vi "DAQX mod 1SDI v04.vi"(0 "resource name":refnum<k15>="PXI1Slot2", 1 "close (T)":bool=TRUE, 2 "Record Data":bool, 3 "numSamples":i32=-1, 4 "max time (s)":dbl=10.0 caption="max time", 5 "min sample rate":dbl=100000000.0, 6 "File location":path, 7 "error in":errorcluster, 8 "reference position":dbl=50.0, 9 "Additional text":string, 10 "Type of measurement":T2, 11 "Name root":string, 13 "channel parameters":T4(array[cluster])=[{"channel name"="0", "input impedance"=0, "maximum input frequency"=30000000.0, "vertical coupling"=1, "probe attenuation"=1.0, "vertical range"=2.0, "vertical offset"=0.0, "channel enabled"=TRUE}, {"channel name"="1", "input impedance"=0, "maximum input frequency"=30000000.0, "vertical coupling"=1, "probe attenuation"=1.0, "vertical range"=2.0, "vertical offset"=0.0, "channel enabled"=TRUE}] {"input impedance" items=["1 mega ohm"=0, "50 ohms"=2]; "vertical coupling" items=["AC", "DC", "Ground"]}, 15 "reset sn":bool) -> (18 "wfm out":waveform(dbl)[](array[waveform]), 22 "Parameters values file":string, 24 "actualSamples 0":i32, 26 "actualSamples 1":i32, 27 "error out":errorcluster caption="error out final")   [LabVIEW 2013]
doc: "Configures and acquires data from an NI-SCOPE high-speed digitizer.\n--------------------\n\nThis Express VI is configured as follows:\n\nDevice: PXI1Slot2 (PXI-5122)\nSample Rate (S/s): 100M\nRecord length: 2k\nAcquisition Mode: N Samples\nChannel 0\n - Range (V): 2\n - Offset (V): 0\n - Probe attenuation: 1\n - Coupling: \n - Input impedence: 1 \n - Bandwidth (Hz): 0\nChannel 1\n - Range (V): 2\n - Offset (V): 0\n - Probe attenuation: 1\n - Coupling: \n - Input impedence: 1 \n - Bandwidth (Hz): 0\nImmediate"
uses:
  <instrlib>/niScope/Controls/niScope vertical coupling.ctl
  Strict Type Defs/type_meas_enum.ctl
  <instrlib>/niScope/Controls/niScope timestamp type.ctl
  Global VIs/shotnoise.vi
  <instrlib>/niScope/Configure/Trigger/niScope Configure Trigger Immediate.vi
  <instrlib>/niScope/Acquire/Fetch/niScope Multi Fetch Binary 16.vi
  <instrlib>/niScope/Acquire/Fetch/niScope Multi Fetch WDT.vi
panel:
  out "Numeric":i32
  out "acquisition status":i32 caption="集録ステータス"
  out "Chan 1 params":T1
  out "Chan 0 params":T1
  out "file location into parameter files":path
  out "size(s)":i32
  out "actual sample rate":dbl
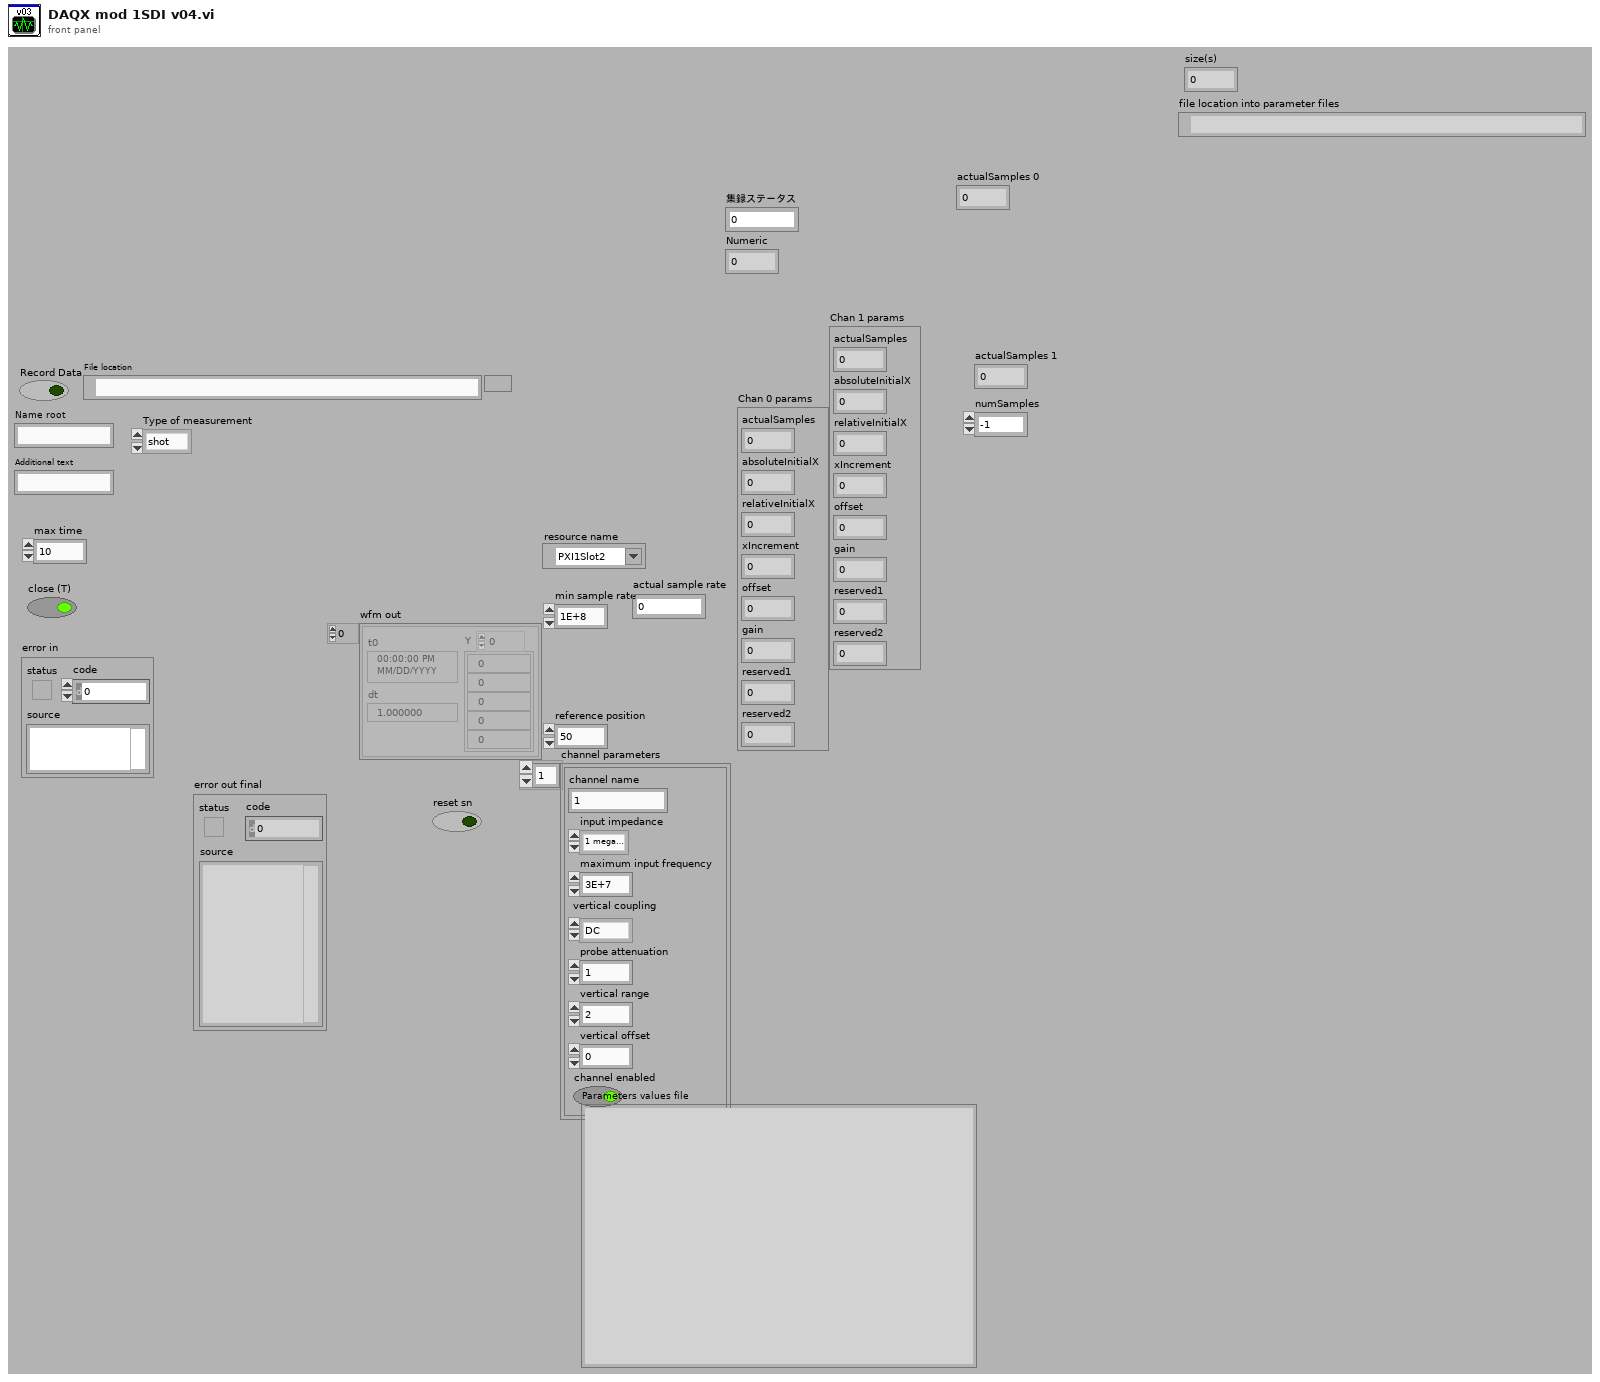
[diagram p1: front panel]
types:
  T1 = cluster{"actualSamples":i32, "absoluteInitialX":dbl, "relativeInitialX":dbl, "xIncrement":dbl, "offset":dbl, "gain":dbl, "reserved1":dbl, "reserved2":dbl}
  T2 = typedef "type_meas_enum.ctl" = enum16{"shot", "x", "p", "electronic"}
  T3 = typedef "niScope vertical coupling.ctl" = i32
  T4 = cluster{"channel name":string, "input impedance":u32, "maximum input frequency":dbl, "vertical coupling":T3, "probe attenuation":dbl, "vertical range":dbl, "vertical offset":dbl, "channel enabled":bool}[]
  T5 = typedef "niScope timestamp type.ctl" = i32
  T6 = cluster{"actualSamples":i32, "absoluteInitialX":dbl, "relativeInitialX":dbl, "xIncrement":dbl, "offset":dbl, "gain":dbl, "reserved1":dbl, "reserved2":dbl}[]
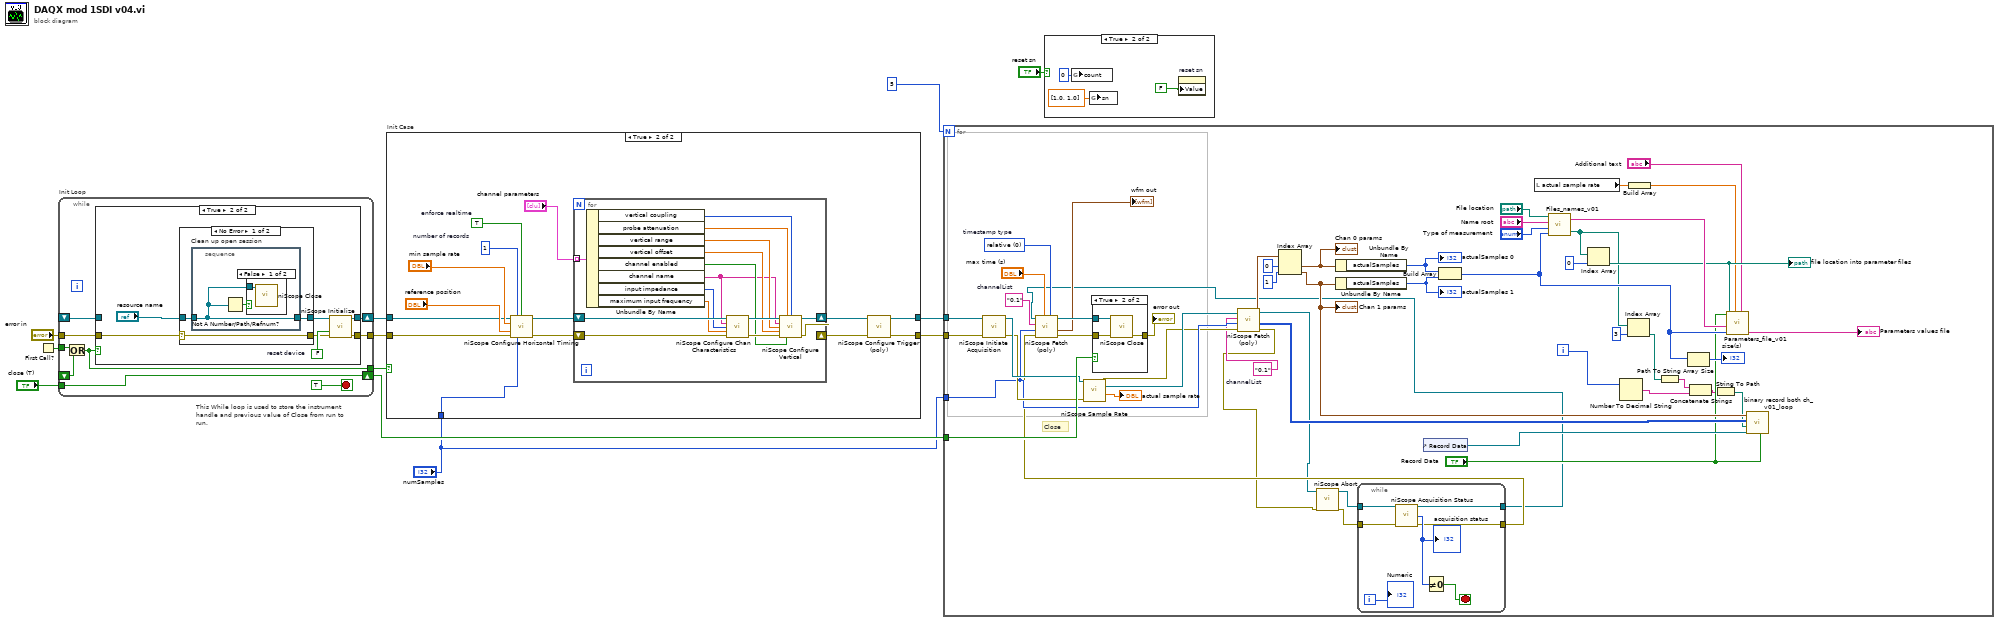
[diagram p0: block diagram]
diagram:
  # "This While loop is used to store the instrument handle and previous value of Close from run to run."
  n1 = First Call?() -> (First Call?: T/F=w10:bool)
  n2 = while "Init Loop" {
    tunnel: w10 -> [w21]
    shift-right: [w20] -> w6
    shift-left: _ -> [w17]
    tunnel: "close (T)" -> [w20]
    shift-right: [w19] -> w9
    shift-left: _ -> [w18]
    tunnel: [w15] -> w8
    tunnel: "error in" -> [w14]
    tunnel: [w13] -> w7
    stop <- TRUE ("stopInit") stop-if-true
    n3 = Or(x=w21, y=w17) -> (x .or. y?=w13:bool)
    n4 = case "Select_Init" shown="True" w13 {
      tunnel: [w23 w28] -> w19
      tunnel: w18 -> [w23 _]
      tunnel: [w22 w27] -> w15
      tunnel: w14 -> [w22 w26]
      frame False {
      }
      frame True {
        w29 = FALSE  # reset device
        n5 = case shown="No Error" w26 {
          selector: w26 -> [w31 w37]
          tunnel: [w33 w38] -> w30
          tunnel: "resource name" -> [w32 w38]
          tunnel: [w31 w37] -> w25
          frame No Error {
            n6 = stacked-sequence "Clean up open session" {
              tunnel: w32 -> [w34]
              tunnel: [w34] -> w33
              frame #0 {
                n7 = Not A Number/Path/Refnum?(number/path/refnum=w34) -> (NaN/Path/Refnum?=w35:bool)
                n8 = case shown="False" w35 {
                  tunnel: w34 -> [w36 _]
                  frame False {
                    n9 = call <instrlib>:"niScope Close.vi"("instrument handle"=w36) -> ()  [unwired: 1 in, 14 out]
                  }
                  frame True {
                  }
                }
              }
            }
          }
          frame Error {
          }
        }
        n10 = call <instrlib>:"niScope Initialize.vi"("resource name"=w30, "reset device"=w29, "error in"=w25) -> ("instrument handle"=w28:refnum<k15>, "error out"=w27:errorcluster)  [unwired: 2 in, 9 out]
      }
    }
  }
  n11 = case "Init Case" shown="True" w7 {
    tunnel: w8 -> [w39 w45]
    tunnel: [w39 w47] -> w12
    tunnel: [w40 w48] -> w11
    tunnel: w9 -> [w40 w46]
    tunnel: "numSamples" -> [_ w41]
    frame False {
    }
    frame True {
      w53 = 1  # number of records
      w54 = TRUE  # enforce realtime
      n12 = call <instrlib>:"niScope Configure Horizontal Timing.vi"("instrument handle"=w46, "number of records"=w53, "enforce realtime"=w54, "min sample rate"="min sample rate", "reference position"="reference position", "error in"=w45, "min record length"=w41) -> ("instrument handle out"=w49:refnum<k15>, "error out"=w50:errorcluster)  [unwired: 7 out]
      n13 = for {
        shift-right: [w57] -> w42
        shift-left: w50 -> [w69]
        shift-right: [w56] -> w43
        shift-left: w49 -> [w68]
        tunnel: "channel parameters" -> [w65] mode=indexing
        n14 = Unbundle By Name(w65) -> ("vertical coupling"=w62:T3, "probe attenuation"=w61:dbl, "vertical range"=w60:dbl, "vertical offset"=w59:dbl, "channel enabled"=w58:bool, "channel name"=w55:string, "input impedance"=w63:u32, "maximum input frequency"=w64:dbl)
        n15 = call <instrlib>:"niScope Configure Chan Characteristics.vi"("instrument handle"=w68, "channels"=w55, "input impedance"=w63, "maximum input frequency"=w64, "error in"=w69) -> ("instrument handle out"=w67:refnum<k15>, "error out"=w66:errorcluster)  [unwired: 9 out]
        n16 = call <instrlib>:"niScope Configure Vertical.vi"("instrument handle"=w67, "probe attenuation"=w61, "vertical coupling"=w62, "channels"=w55, "vertical range"=w60, "vertical offset"=w59, "error in"=w66, "channel enabled"=w58) -> ("instrument handle out"=w56:refnum<k15>, "error out"=w57:errorcluster)  [unwired: 6 out]
      }
      n17 = call-poly <instrlib>:"niScope Configure Trigger (poly).vi"("instrument handle"=w43, "error in"=w42) -> ("instrument handle out"=w48:refnum<k15>, "error out"=w47:errorcluster)  [unwired: 12 out]
    }
  }
  n18 = for {
    N: 5 -> [_]
    tunnel: w12 -> [w119]
    tunnel: w11 -> [w118]
    tunnel: w6 -> [w116]
    tunnel: "numSamples" -> [w111]
    i -> [w76]
    w92 = "0,1"  # channelList
    w117 = T5 0 items=["relative", "absolute"]  # timestamp type
    w120 = "0,1"  # channelList
    # "Close"
    n19 = call <instrlib>:"niScope Initiate Acquisition.vi"("instrument handle"=w118, "error in"=w119) -> ("instrument handle out"=w114:refnum<k15>, "error out"=w113:errorcluster)  [unwired: 12 out]
    n20 = call <instrlib>:"niScope Sample Rate.vi"("instrument handle"=w114, "error in"=w113) -> ("instrument handle out"=w110:refnum<k15>, "actual sample rate"=→"actual sample rate":dbl, "error out"=w109:errorcluster)  [unwired: 11 out]
    n21 = call-poly <instrlib>:"niScope Fetch (poly).vi"("error in"=w109, "numSamples"=w111, "channels"=w92, "instrument handle"=w110) -> ("error out"=w71:errorcluster, "wfm"=w86:i16[][], "wfm info"=w108:T6, "instrument handle out"=w73:refnum<k15>)  [unwired: 1 in, 3 out]
    n22 = Index Array(array=w108, index #1=0 ("index"), index #2=1 ("index")) -> (element #1=w105:T1, element #2=w87:T1)
    "Chan 0 params" <- w105
    "Chan 1 params" <- w87
    n23 = call <instrlib>:"niScope Abort.vi"("instrument handle"=w73, "error in"=w71) -> ("instrument handle out"=w72:refnum<k15>, "error out"=w70:errorcluster)  [unwired: 12 in]
    n24 = Unbundle By Name(w105) -> ("actualSamples"=w104:i32)
    "actualSamples 0" <- w104
    n25 = Unbundle By Name(w87) -> ("actualSamples"=w89:i32)
    "actualSamples 1" <- w89
    n26 = while {
      tunnel: w72 -> [w129]
      tunnel: w70 -> [w128]
      tunnel: [w125] -> w75
      tunnel: [w124] -> w74
      i -> [w123]
      stop <- w126 stop-if-true
      n27 = call <instrlib>:"niScope Acquisition Status.vi"("instrument handle"=w129, "error in"=w128) -> ("instrument handle out"=w124:refnum<k15>, "acquisition status"=w127:i32, "error out"=w125:errorcluster)  [unwired: 11 in]
      "acquisition status" <- w127
      n28 = Not Equal To 0?(x=w127) -> (x != 0?=w126:bool)
      "Numeric" <- w123
    }
    n29 = call-poly <instrlib>:"niScope Fetch (poly).vi"("timestamp Type"=w117, "timeout"="max time (s)", "error in"=w75, "numSamples"=w111, "channels"=w120, "instrument handle"=w74) -> ("error out"=w91:errorcluster, "wfm"=→"wfm out":waveform(dbl)[], "instrument handle out"=w112:refnum<k15>)  [unwired: 3 out]
    n30 = case shown="True" w116 {
      tunnel: w91 -> [w130 w133]
      tunnel: [w130 w132] -> w122
      tunnel: w112 -> [_ w131]
      frame False {
      }
      frame True {
        n31 = call <instrlib>:"niScope Close.vi"("instrument handle"=w131, "error in"=w133) -> ("error out"=w132:errorcluster)  [unwired: 13 out]
      }
    }
    "error out" <- w122
    n32 = control-ref of="Record Data"() -> (w88:refnum<vi>)
    n33 = Build Array(w104, w89) -> (w94:i32[])
    n34 = local read "actual sample rate"() -> (w96:dbl)
    n35 = call "Files_names_v01.vi"("actualSamples\narray"=w94, "Type of\nmeasurement"="Type of measurement", "Name root"="Name root", "File location"="File location") -> ("Files path array"=w83:path[], "Files name array"=w100:string[])
    n36 = Index Array(array=w83, index=0) -> (element=w98:path)
    "file location into parameter files" <- w98
    n37 = Number To Decimal String(number=w76) -> (decimal integer string=w80:string)  [unwired: 1 out]
    n38 = Index Array(array=w83, index=3) -> (element=w81:path)
    n39 = Build Array(w96) -> (w95:dbl[])
    n40 = Path To String(path=w81) -> (string=w79:string)
    n41 = Array Size(array=w94) -> (size(s)=→"size(s)":i32)
    n42 = Concatenate Strings(w79, w80) -> (w78:string)
    n43 = String To Path(string=w78) -> (path=w77:path)
    n44 = call "Parameters_file_v01.vi"("Additional text"="Additional text", "actual sample rate array"=w95, "actualSamples array"=w94, "Files name array"=w100, "File location"=w98, "Record"="Record Data") -> ("Full text"=→"Parameters values file":string)  [unwired: 3 in]
    n45 = call "binary record both ch_v01_loop.vi"("Record"="Record Data", "reference"=w88, "path"=w77, "wfm"=w86, "Chan 1 params"=w87) -> ()  [unwired: 7 in]
  }
  n46 = case shown="True" "reset sn" {
    frame False {
    }
    frame True {
      n47 = global write "shotnoise.vi" "count"(i64 0 ("count")) -> ()
      n48 = global write "shotnoise.vi" "sn"(dbl[] [1.0, 1.0] ("sn")) -> ()
      n49 = property on="reset sn" class="Bool (strict)"("Value"=FALSE ("reset sn")) -> ()  [unwired: 2 in, 2 out]
    }
  }
